vi "Read channel pointer.vi"(8 "error in (no error)":errorcluster, 11 "Runtime.Channel in":refnum<class "Runtime.Channel.lvclass">) -> (0 "error out":errorcluster, 2 "channel pointer":u64 format="%.0x", 3 "Runtime.Channel out":refnum<class "Runtime.Channel.lvclass">)   [LabVIEW 2016, in "Data Sharing Framework.Runtime.lvlib" / "Runtime.Channel.lvclass"]
uses:
  Runtime.Channel.lvclass
  Runtime.Channel.lvclass/Runtime.Channel.ctl
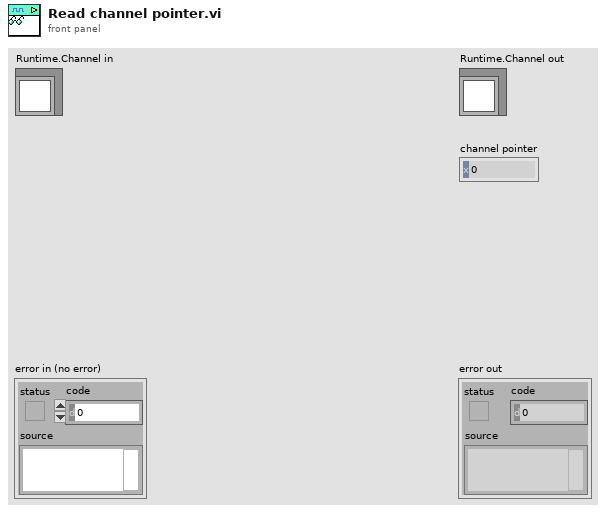
[diagram p1: front panel]
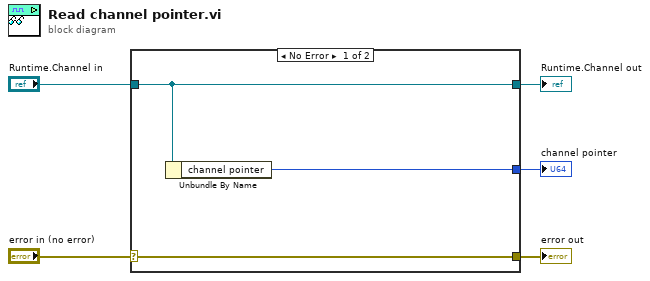
[diagram p0: block diagram]
diagram:
  n1 = case shown="No Error" "error in (no error)" {
    selector: "error in (no error)" -> [w8 w9]
    tunnel: [w8 w9] -> w4
    tunnel: [w7 w10] -> w2
    tunnel: "Runtime.Channel in" -> [w7 w10]
    tunnel: [w6 _] -> w1
    frame No Error {
      n2 = Unbundle By Name(w7) -> ("channel pointer"=w6:u64)
    }
    frame Error {
    }
  }
  "error out" <- w4
  "Runtime.Channel out" <- w2
  "channel pointer" <- w1
